vi "scripting_build_polymorphic_VIs.vi"() -> ()   [LabVIEW 2020]
panel:
  out "Numeric":i32
  out "concatenated string":string
  out "InstanceInfo":T1(array[cluster])
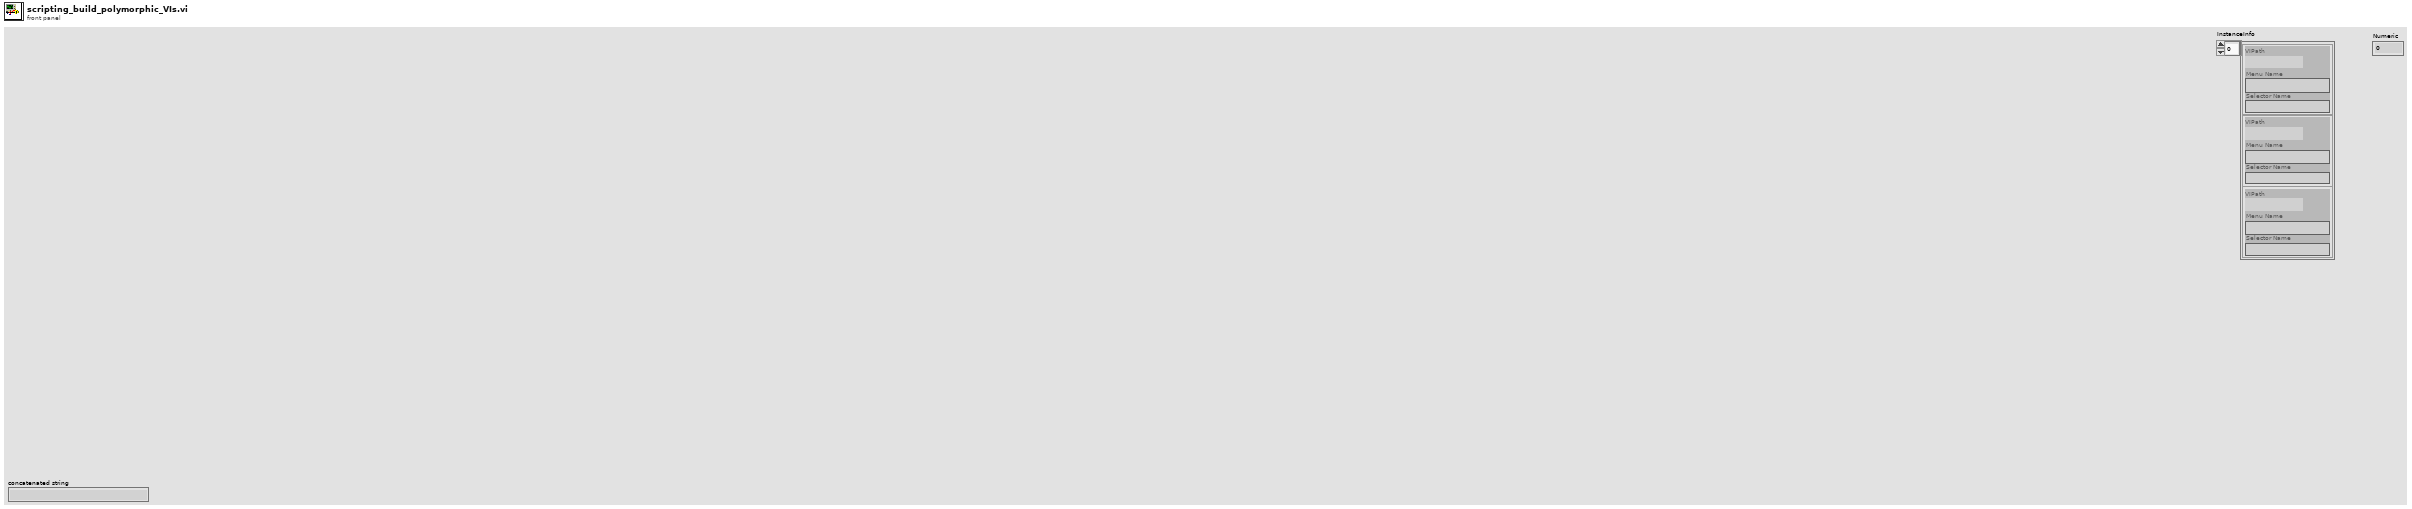
[diagram p1: front panel]
types:
  T1 = cluster{"VIPath":path, "Menu Name":string, "Selector Name":string}[]
  T2 = cluster{"VIPath":path, "Menu Name":string, "Selector Name":string}
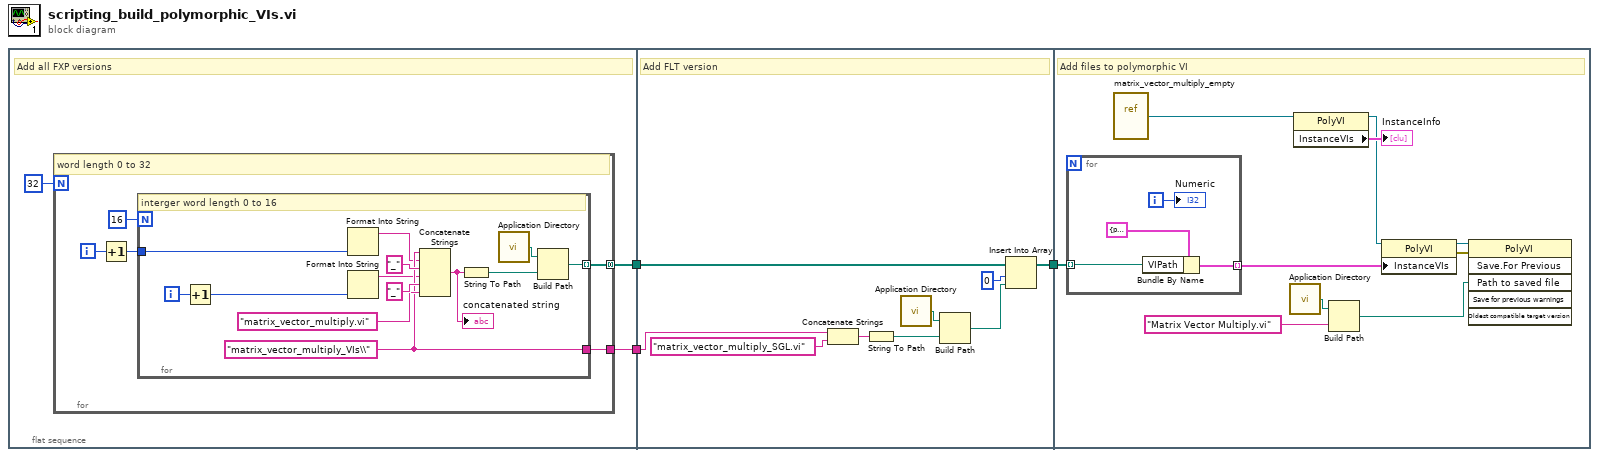
[diagram p0: block diagram]
diagram:
  n1 = flat-sequence {
    tunnel: [w5] -> w2
    tunnel: [w4] -> w1
    tunnel: [w26] -> w3
    tunnel: w2 -> [w27]
    tunnel: w1 -> [w25]
    tunnel: w3 -> [w35]
    frame #0 {
      # "Add all FXP versions"
      n2 = for {
        N: 32 -> [_]
        tunnel: [w8] -> w5 mode=concatenating
        tunnel: [w7] -> w4
        i -> [w11]
        # "word length 0 to 32"
        n3 = Increment(x=w11) -> (x+1=w9:i32)
        n4 = for {
          N: 16 -> [_]
          tunnel: w9 -> [w24]
          tunnel: [w15] -> w8 mode=indexing
          tunnel: [w14] -> w7
          i -> [w22]
          w14 = "matrix_vector_multiply_VIs\\" ("string")
          # "interger word length 0 to 16"
          n5 = Increment(x=w22) -> (x+1=w23:i32)
          n6 = Format Into String(w24) -> (resulting string=w13:string)  [unwired: 3 in, 1 out]
          n7 = Format Into String(w23) -> (resulting string=w12:string)  [unwired: 3 in, 1 out]
          n8 = Concatenate Strings(w14, w13, "_" ("string"), w12, "_" ("string"), "matrix_vector_multiply.vi" ("string")) -> (w16:string)
          "concatenated string" <- w16
          n9 = String To Path(string=w16) -> (path=w21:path)
          n10 = call <vilib>:"Application Directory.vi"() -> ("Application Directory"=w20:path)
          n11 = Build Path(base path=w20, name or relative path=w21) -> (appended path=w15:path)
        }
      }
    }
    frame #1 {
      # "Add FLT version"
      n12 = Concatenate Strings(w25, "matrix_vector_multiply_SGL.vi" ("string")) -> (w32:string)
      n13 = String To Path(string=w32) -> (path=w31:path)
      n14 = call <vilib>:"Application Directory.vi"() -> ("Application Directory"=w30:path)
      n15 = Build Path(base path=w30, name or relative path=w31) -> (appended path=w33:path)
      n16 = Insert Into Array(array=w27, index=0, new element=w33) -> (w26:path[])
    }
    frame #2 {
      # "Add files to polymorphic VI"
      n17 = for {
        tunnel: [w47] -> w43 mode=indexing
        tunnel: w35 -> [w46] mode=indexing
        i -> [w44]
        n18 = Bundle By Name(cluster=T2 {"VIPath"=path "", "Menu Name"="", "Selector Name"=""}, "VIPath"=w46) -> (w47:T2)
        "Numeric" <- w44
      }
      n19 = vi-ref "matrix_vector_multiply_empty.vi"() -> (w34:refnum<vi>)
      n20 = call <vilib>:"Application Directory.vi"() -> ("Application Directory"=w39:path)
      n21 = property class="PolyVI"(reference=w34) -> (reference out=w41:refnum<vi>, "InstanceVIs"=→"InstanceInfo":T1)  [unwired: 1 in, 1 out]
      n22 = Build Path(base path=w39, name or relative path="Matrix Vector Multiply.vi" ("string")) -> (appended path=w38:path)
      n23 = property class="PolyVI"(reference=w41, "InstanceVIs"=w43) -> (reference out=w37:refnum<vi>, error out=w36:errorcluster)  [unwired: 1 in]
      n24 = invoke class="PolyVI" method="Save.For Previous"(reference=w37, error in=w36, "Path to saved file"=w38) -> ()  [unwired: 3 in, 6 out]
    }
  }
